vi "XandY aimer.vi"(8 "Aiming?":bool, 10 "Distance":dbl, 11 "Image width":dbl) -> (0 "Good enough?":bool, 1 "Y-setpoint":dbl, 3 "X setpoint":dbl, 5 "Aiming?":bool)   [LabVIEW 2015]
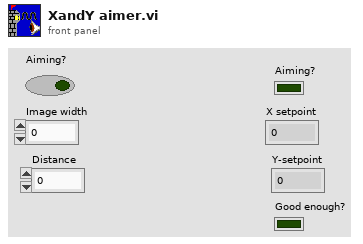
[diagram p1: front panel]
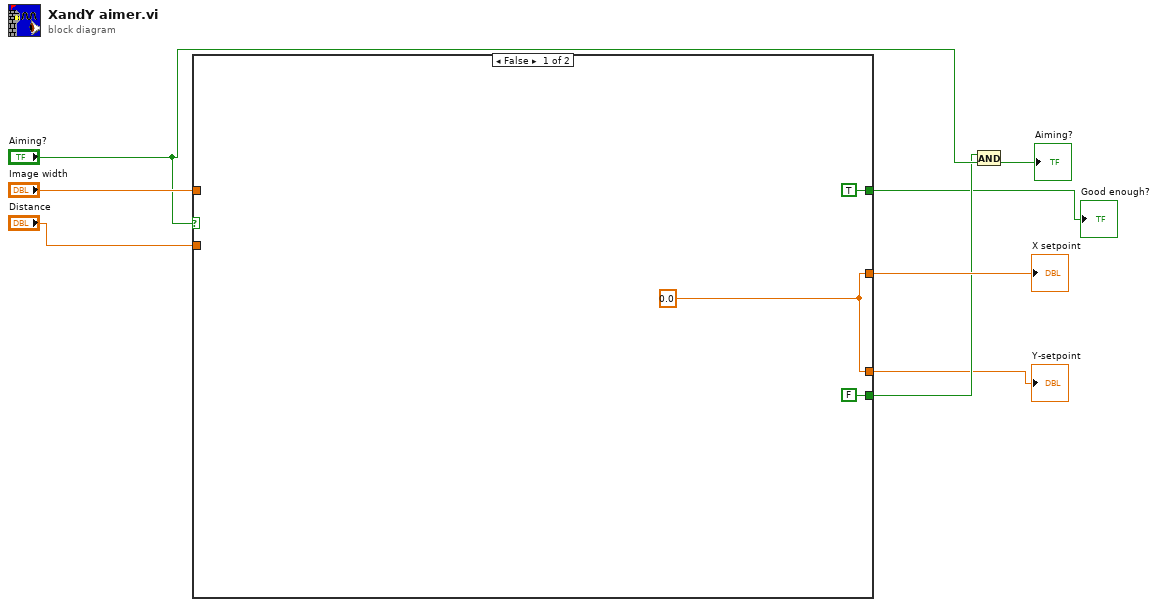
[diagram p0: block diagram]
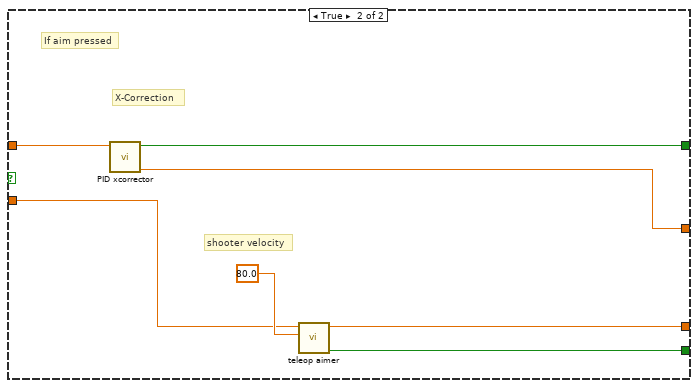
[diagram p2: hidden frame]
diagram:
  n1 = case shown="False" "Aiming?" {
    tunnel: "Image width" -> [_ w17]
    tunnel: "Distance" -> [_ w16]
    tunnel: [w11 w13] -> w5
    tunnel: [FALSE ("Aim Possible?") w15] -> w3
    tunnel: [w11 w14] -> w2
    tunnel: [TRUE ("Good Enough?") w12] -> w1
    frame False {
      w11 = 0.0 ("Motor out")
    }
    frame True {
      # "shooter velocity"
      # "If aim pressed"
      # "X-Correction"
      n2 = call "PID xcorrector.vi"("Image width"=w17) -> ("Motor out"=w13:dbl, "Good Enough?"=w12:bool)  [unwired: 9 in]
      n3 = call "teleop aimer.vi"("velocity"=80.0, "Distance"=w16) -> ("Aim Possible?"=w15:bool, "Target Vert Angle"=w14:dbl)  [unwired: 8 in]
    }
  }
  "X setpoint" <- w5
  "Y-setpoint" <- w2
  "Good enough?" <- w1
  n4 = And(x=w3, y="Aiming?") -> (x .and. y?=→"Aiming?":bool)
